vi "Read Data.vi"(8 "error in (no error)":errorcluster, 11 "Controller in":refnum<class "Controller.lvclass">) -> (0 "error out":errorcluster, 2 "Data":T1, 3 "Controller out":refnum<class "Controller.lvclass">)   [LabVIEW 2014]
uses:
  Controller.lvclass
  reusable/PAS/Data/Main/PAS Data.lvclass
  reusable/CRDS/Data/Main/CRDS Data.lvclass
  Devices/Alicat/Session Based/Data/Alicat Data.lvclass
  reusable/Data/Array Data/Single 1-D/Single_Array.lvclass
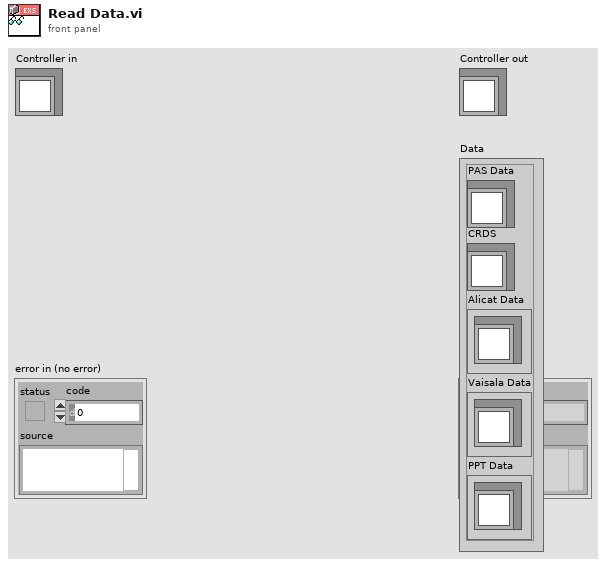
[diagram p1: front panel]
types:
  T1 = cluster{"PAS Data":refnum<class "PAS Data.lvclass">, "CRDS":refnum<class "CRDS Data.lvclass">, "Alicat Data":refnum<class "Alicat Data.lvclass">[], "Vaisala Data":refnum<class "Single_Array.lvclass">[], "PPT Data":refnum<class "Single_Array.lvclass">[]}
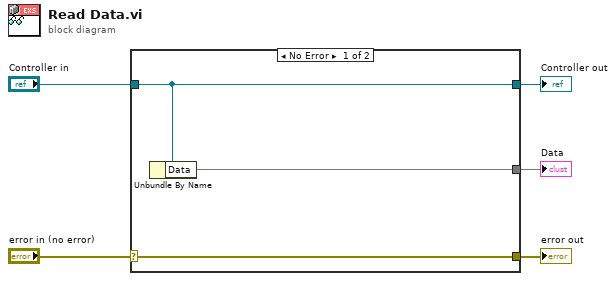
[diagram p0: block diagram]
diagram:
  n1 = case shown="No Error" "error in (no error)" {
    selector: "error in (no error)" -> [w8 w9]
    tunnel: [w8 w9] -> w4
    tunnel: [w7 w10] -> w2
    tunnel: "Controller in" -> [w7 w10]
    tunnel: [w6 _] -> w1
    frame No Error {
      n2 = Unbundle By Name(w7) -> ("Data"=w6)
    }
    frame Error {
    }
  }
  "error out" <- w4
  "Controller out" <- w2
  "Data" <- w1
